vi "TIO SLIP Tests.vi"() -> ()   [LabVIEW 2017]
panel:
  out "Random Test":bool
  out "Random Test":string
  out "Example Test":bool
  # "Try running continuously"
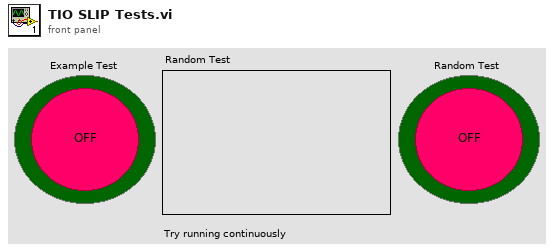
[diagram p1: front panel]
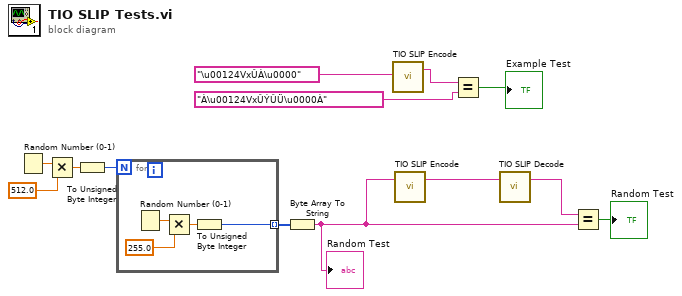
[diagram p0: block diagram]
diagram:
  n1 = Random Number (0-1)() -> (number: 0 to 1=w9:dbl)
  n2 = Multiply(x=w9, y=512.0) -> (x*y=w7:dbl)
  n3 = To Unsigned Byte Integer(number=w7) -> (unsigned 8bit integer=w6:u8)
  n4 = for {
    N: w6 -> [_]
    tunnel: [w14] -> w5 mode=indexing
    n5 = Random Number (0-1)() -> (number: 0 to 1=w17:dbl)
    n6 = Multiply(x=w17, y=255.0) -> (x*y=w15:dbl)
    n7 = To Unsigned Byte Integer(number=w15) -> (unsigned 8bit integer=w14:u8)
  }
  n8 = Byte Array To String(unsigned byte array=w5) -> (string=w2:string)
  "Random Test" <- w2
  n9 = call <instrlib>:"TIO SLIP Encode.vi"("String Input"="\u00124VxÛÀ\u0000") -> ("SLIP Output"=w11:string)  [unwired: 1 in, 1 out]
  n10 = call <instrlib>:"TIO SLIP Encode.vi"("String Input"=w2) -> ("SLIP Output"=w4:string)  [unwired: 1 in, 1 out]
  n11 = Equal?(x=w11, y="À\u00124VxÛÝÛÜ\u0000À" ("SLIP Output")) -> (x = y?=→"Example Test":bool)
  n12 = call <instrlib>:"TIO SLIP Decode.vi"("SLIP Input"=w4) -> ("String Output"=w3:string)  [unwired: 1 in, 1 out]
  n13 = Equal?(x=w3, y=w2) -> (x = y?=→"Random Test":bool)
